vi "ServiceClient.vi"(0 "Topic":string="/junk", 1 "node":string, 2 "Msg in":string="test", 3 "error in":errorcluster) -> (5 "Reply":string, 6 "error out":errorcluster)   [LabVIEW 2016]
doc: "Starts a service client on the RIO"
uses:
  ROS/Code/Console/Servers/ServerSubs/TopicDef.ctl
  ROS/Code/SubVIs/_ROSDirection.ctl
  ROS/MessageBuilding/std_msgs/subs/stringScalar.vi
  ROS/MessageParsing/std_msgs/subs/parse_u8_scalar.vi
  ROS/MessageParsing/std_msgs/subs/parse_string_scalar.vi
panel:
  out "Original reply":string
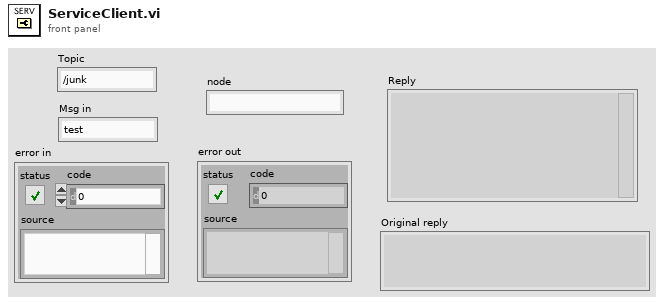
[diagram p1: front panel]
types:
  T1 = typedef "TopicDef.ctl" = cluster{"Topic":string, "Type":string, "Action":T2, "Update (ms)":u16, "queue size":u16}
  T2 = typedef "_ROSDirection.ctl" = enum16{"Node", "Publisher", "Subscriber", "ServiceClient", "ServiceProvider"}
  T3 = typedef "_ROSControl.ctl" = cluster{"topic port":u16, "Node":string, "topic":string, "type":string, "node port":u16, "error ":errorcluster, "Direction":T2, "Update (ms)":u16, "FIFO size":u16}
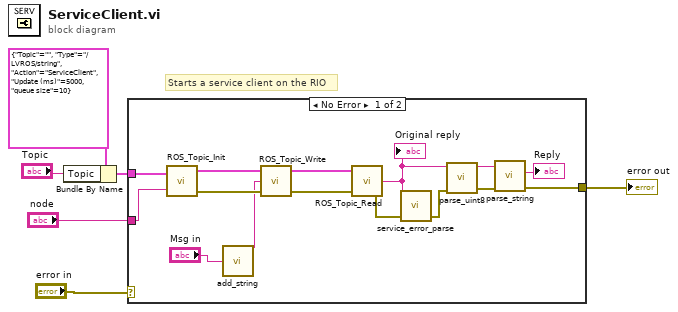
[diagram p0: block diagram]
diagram:
  # "Starts a service client on the RIO"
  n1 = Bundle By Name(cluster=T1 {"Topic"="", "Type"="/LVROS/string", "Action"=enum."ServiceClient", "Update (ms)"=5000, "queue size"=10} ("Definitions"), "Topic"="Topic") -> (w3:T1)
  n2 = case shown="No Error" "error in" {
    selector: "error in" -> [_ w22]
    tunnel: "node" -> [w21 _]
    tunnel: w3 -> [w20 _]
    tunnel: [w9 w22] -> w2
    frame No Error {
      n3 = call "ROS_Topic_Init.vi"("Definitions"=w20, "node"=w21) -> ("ROS out"=w8:T3, "error out"=w18:errorcluster)  [unwired: 1 in]
      n4 = call-poly "add_string.vi"("String"="Msg in") -> ("msg out"=w15:string)  [unwired: 4 in]
      n5 = call "ROS_Topic_Write.vi"("error in (no error)"=w18, "Msg in"=w15, "ROS in"=w8) -> ("error out"=w17:errorcluster, "ROS out"=w7:T3)  [unwired: 1 in]
      n6 = call "ROS_Topic_Read.vi"("error in (no error)"=w17, "ROS in"=w7) -> ("error out"=w16:errorcluster, "Reply"=w14:string)  [unwired: 1 in, 1 out]
      "Original reply" <- w14
      n7 = call "service_error_parse.vi"("error in (no error)"=w16, "Reply"=w14) -> ("error out"=w11:errorcluster)  [unwired: 1 in, 2 out]
      n8 = call-poly "parse_uint8.vi"("error in"=w11, "msg in"=w14) -> ("error out"=w10:errorcluster, "msg out"=w13:string)  [unwired: 3 in, 1 out]
      n9 = call-poly "parse_string.vi"("error in"=w10, "msg in"=w13) -> ("error out"=w9:errorcluster, "string"=→"Reply":string)  [unwired: 3 in, 1 out]
    }
    frame Error {
    }
  }
  "error out" <- w2
